vi "Stream to Image Files.vi"() -> ()   [LabVIEW 2023]
doc: "The Stream to Image Files example shows how to save images to PNG files in parallel when using a grab acquisition. Images acquired from a camera are stored in a manager and each worker loop removes an image from the manager to save to disk. When the save to disk is complete, the image is added back to the manager so it can be used to copy acquired images into again. It is recommended to use the Stream to Image Files (Optimized Performance) example if your camera settings work with a ring acquisition."
uses:
  SubVIs/Grab Manager Mode.ctl
  <vilib>/vision/driver/IMAQdx.llb/IMAQdx Buffer Number Mode.ctl
  <vilib>/Utility/High Resolution Relative Seconds.vi
  <vilib>/vision/driver/NI_Vision_Acquisition_Software.lvlib
  <resource>/objmgr/imaqdx.rc
panel:
  out "Images Acquired Per Second":dbl
  in  "Skip Count":u32
  in  "Number of Workers":u8=3 min=1 max=3
  out "Images Behind":i32
  out "Images Saved Per Second":dbl
  in  "Number of Images":u32=30
  out "Destination Folder":path
  out "Write Speed":dbl(graph) caption="Image File Write Speed"
  in  "Camera Name":refnum<k21> caption="IMAQdx Session"
  in  "Stop":bool
  # "Overview: Demonstrates how to stream images to disk in parallel when using a ring acquisition.\nRequirements: Vision Acquisition Software\nInstructions:\n1. Select the Camera Name\n2. Run the VI\n3. Reduce the Number of Workers to see if the streaming of images can keep up with fewer workers.\n4. Increase the Skip Count if Images Behind is greater than 0."
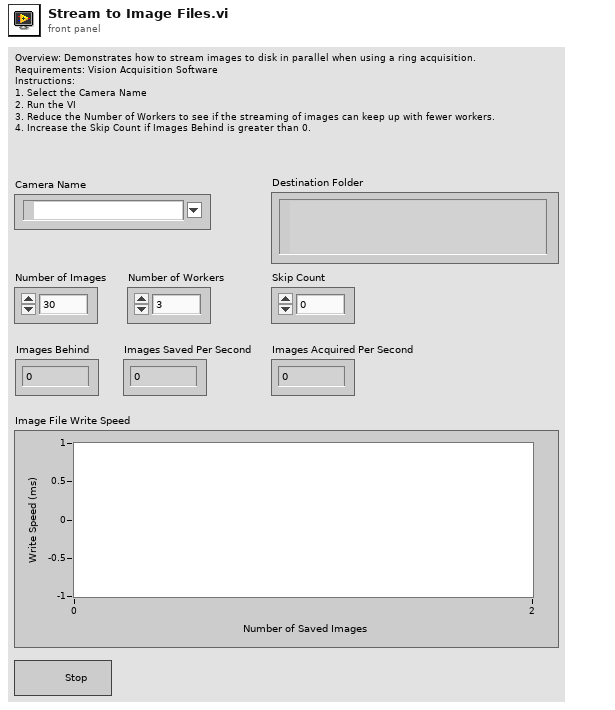
[diagram p1: front panel]
types:
  T1 = cluster{"Number of Processing Images":u32, "Image Border Size":u32}
  T2 = typedef "Grab Manager Mode.ctl" = enum16{"Create Processing Images", "Lock", "Add Acquired Image", "Get Acquired Image", "Unlock", "Dispose Processing Images"}
  T3 = typedef "IMAQdx.ctl" = refnum<k21>
  T4 = typedef "NI_Vision_Acquisition_Software.lvlib/IMAQdx Buffer Number Mode.ctl" = enum32{"Next", "Last", "Buffer Number", "Every", "Last New"}
  T5 = typedef "IMAQ Image.ctl" = refnum<image>
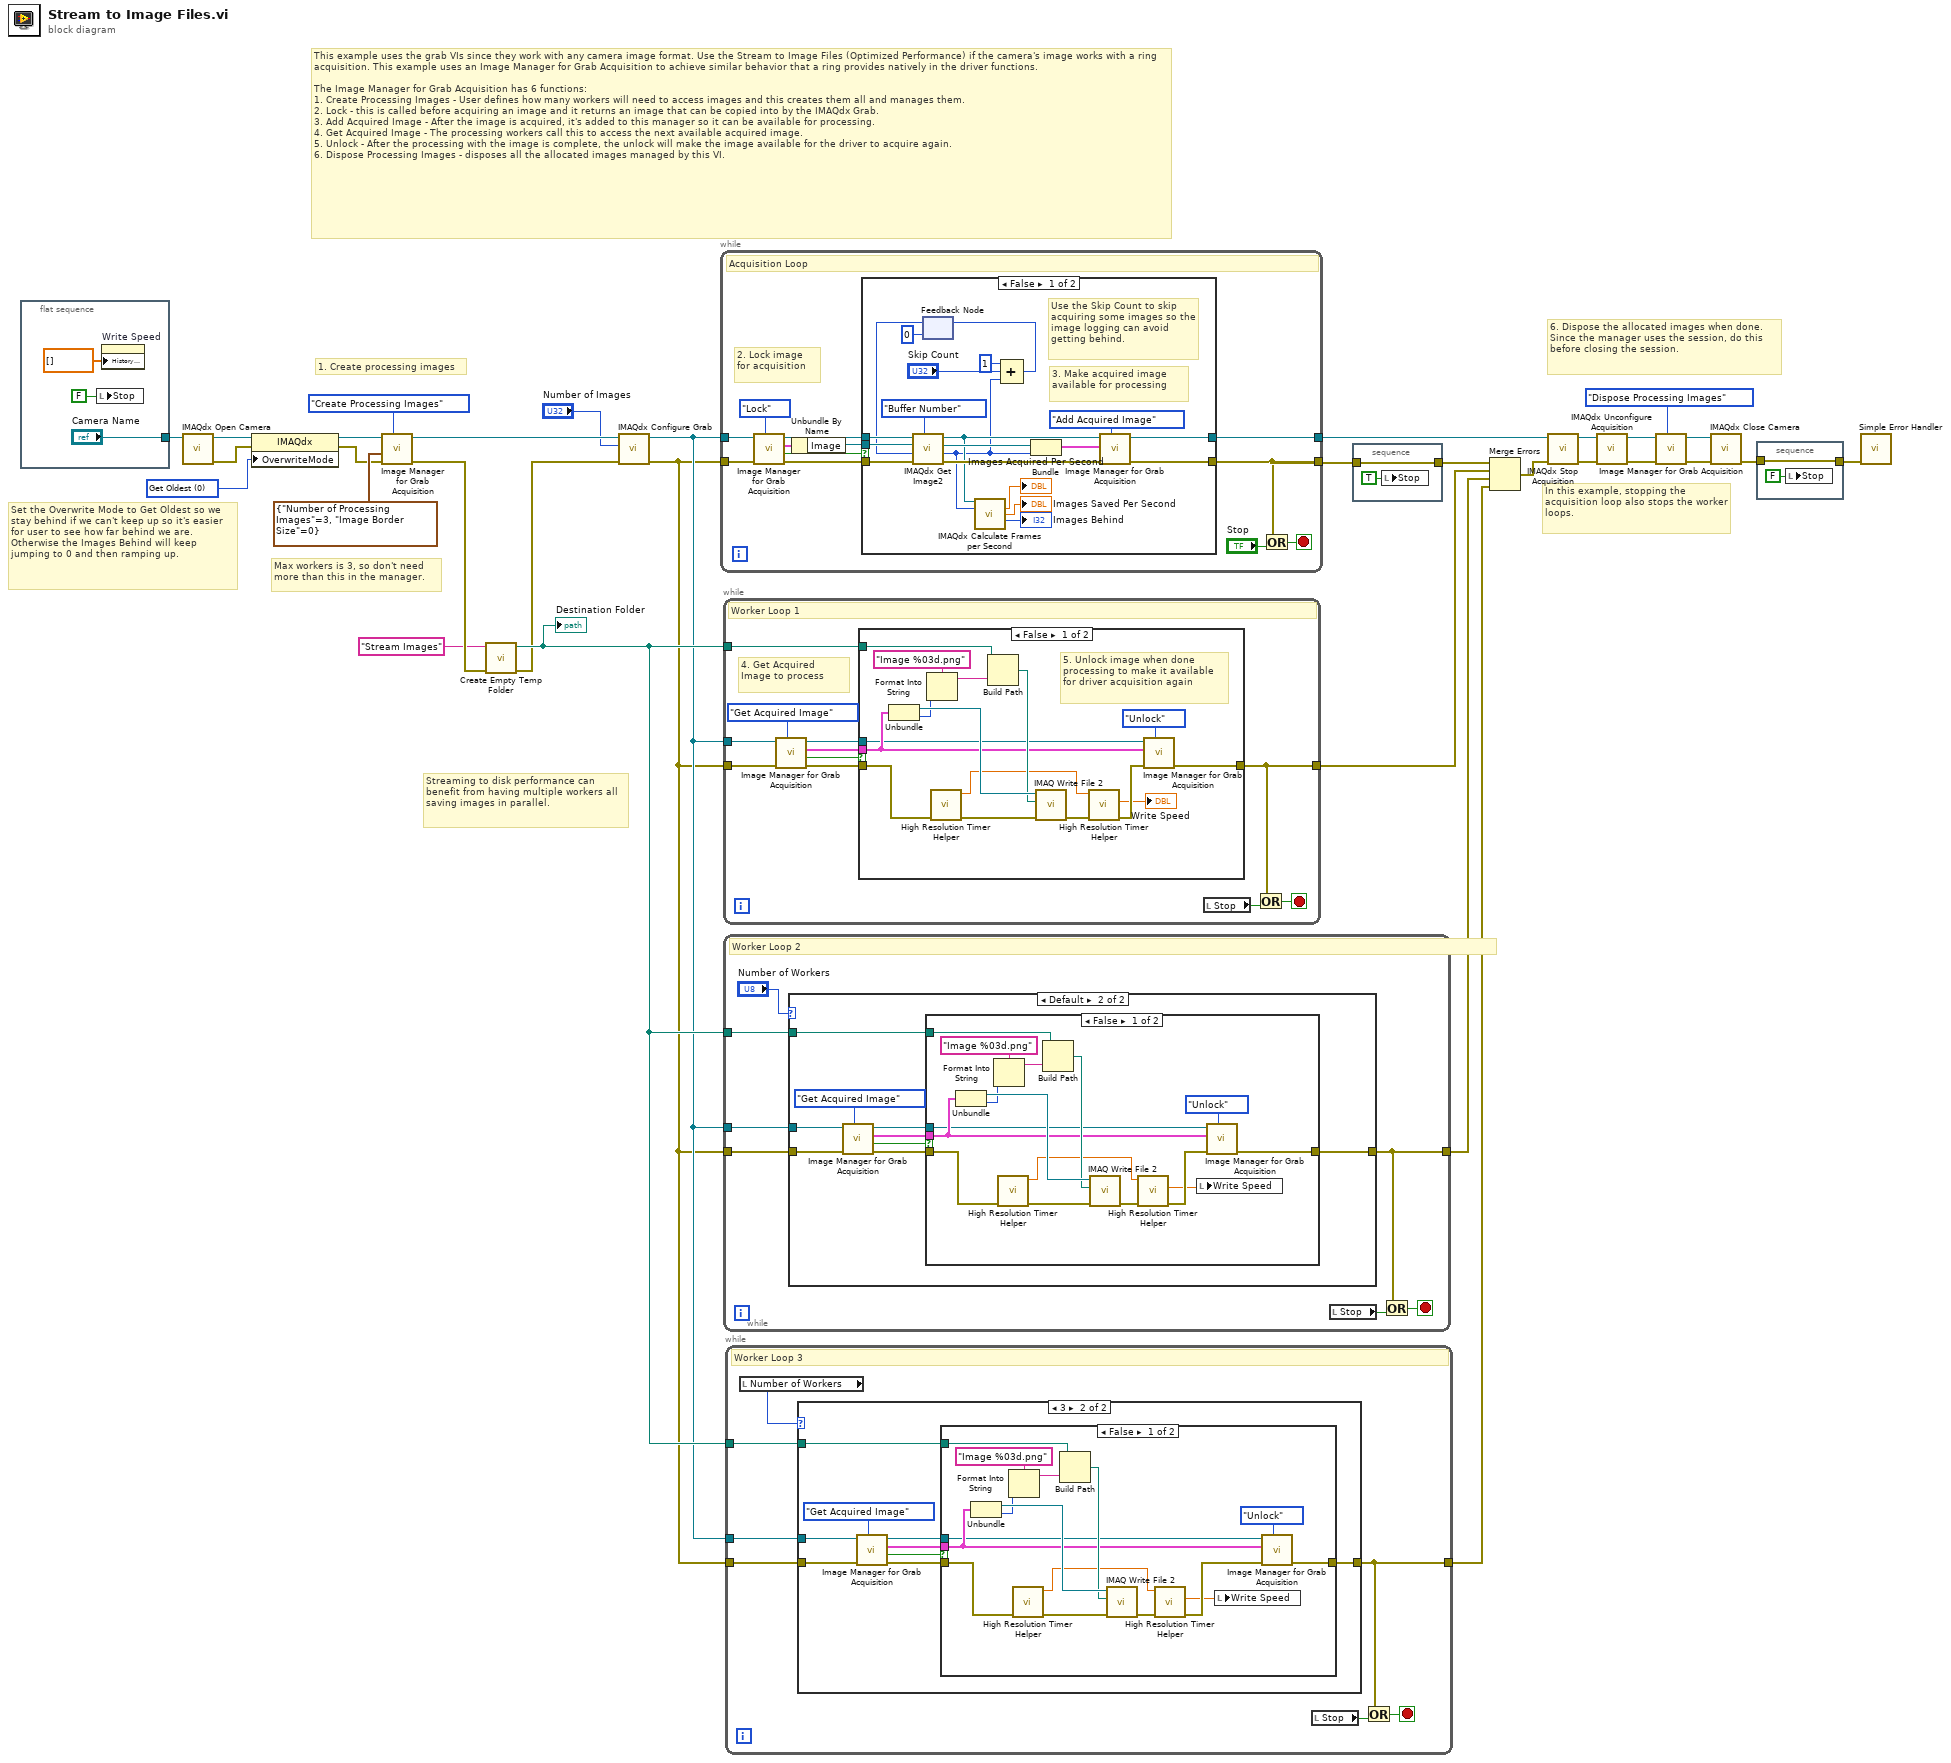
[diagram p0: block diagram]
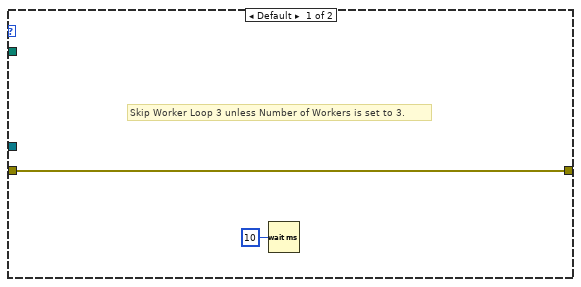
[diagram p2: hidden frame]
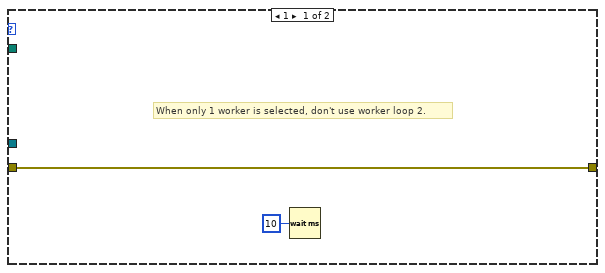
[diagram p4: hidden frame]
diagram:
  w19 = u32 0 items=["Get Oldest"=0, "Fail"=2, "Get Newest"=3] ("OverwriteMode")
  # "6. Dispose the allocated images when done. Since the manager uses the session, do this before closing the session."
  # "1. Create processing images"
  # "This example uses the grab VIs since they work with any camera image format. Use the Stream to Image Files (Optimized Performance) if the camera's image works with a ring acquisition. This example uses an Image Manager for Grab Acquisition to achieve similar behavior that a ring provides natively in the driver functions.\n\nThe Image Manager for Grab Acquisition has 6 functions:\n1. Create Processing Images - User defines how many workers will need to access images and this creates them all and manages them.\n2. Lock - this is called before acquiring an image and it returns an image that can be copied into by the IMAQdx Grab.\n3. Add Acquired Image - After the image is acquired, it's added to this manager so it can be available for processing.\n4. Get Acquired Image - The processing workers call this to access the next available acquired image.\n5. Unlock - After the processing with the image is complete, the unlock will make the image available for the driver to acquire again.\n6. Dispose Processing Images - disposes all the allocated images managed by this VI."
  # "Set the Overwrite Mode to Get Oldest so we stay behind if we can't keep up so it's easier for user to see how far behind we are. Otherwise the Images Behind will keep jumping to 0 and then ramping up."
  # "Max workers is 3, so don't need more than this in the manager."
  # "In this example, stopping the acquisition loop also stops the worker loops."
  # "Streaming to disk performance can benefit from having multiple workers all saving images in parallel."
  n1 = flat-sequence {
    tunnel: ["Camera Name"] -> w32
    frame #0 {
      n2 = local write "Stop"(FALSE ("Stop")) -> ()
      n3 = property on="Write Speed" class="WFChart (strict)"("History Data"=dbl[] []) -> ()  [unwired: 2 in, 2 out]
    }
  }
  n4 = call <vilib>:"IMAQdx Open Camera.vi"("Session In"=w32) -> ("error out"=w10:errorcluster, "Session Out"=w20:T3)  [unwired: 2 in, 7 out]
  n5 = property class="IMAQdx"(reference=w20, error in=w10, "OverwriteMode"=w19) -> (reference out=w9:T3, error out=w8:errorcluster)
  n6 = call "Image Manager for Grab Acquisition.vi"("Mode"=Grab_Manager_Mode."Create Processing Images", "error in (no error)"=w8, "Init Settings"=T1 {"Number of Processing Images"=3, "Image Border Size"=0}, "Session In"=w9) -> ("error out"=w7:errorcluster, "Session Out"=w5:T3)  [unwired: 4 in, 2 out]
  n7 = call "Create Empty Temp Folder.vi"("error in (no error)"=w7, "Folder Name"="Stream Images") -> ("error out"=w4:errorcluster, "Empty Temp Folder"=w22:path)  [unwired: 8 in]
  "Destination Folder" <- w22
  n8 = call <vilib>:"IMAQdx Configure Grab.vi"("error in"=w4, "Number of Buffers"="Number of Images", "Session In"=w5) -> ("error out"=w2:errorcluster, "Session Out"=w3:T3)  [unwired: 7 in]
  n9 = while {
    tunnel: w2 -> [w45]
    tunnel: w3 -> [w42]
    tunnel: [w43] -> w28
    tunnel: [w44] -> w27
    stop <- w46 stop-if-true
    # "2. Lock image for acquisition"
    # "Acquisition Loop"
    n10 = call "Image Manager for Grab Acquisition.vi"("Mode"=Grab_Manager_Mode."Lock", "error in (no error)"=w45, "Session In"=w42) -> ("error out"=w38:errorcluster, "No Available Image"=w39:bool, "Image Settings Out"=w37:cluster{"Image":T5, "Buffer Number":u32}, "Session Out"=w40:T3)  [unwired: 5 in]
    n11 = Unbundle By Name(w37) -> ("Image"=w36:T5)
    n12 = case shown="False" w39 {
      tunnel: [w59 w69] -> w43
      tunnel: [w58 w68] -> w44
      tunnel: w40 -> [w67 w69]
      tunnel: w38 -> [w66 w68]
      tunnel: w36 -> [w60 _]
      frame False {
        # "3. Make acquired image available for processing"
        # "Use the Skip Count to skip acquiring some images so the image logging can avoid getting behind."
        n13 = feedback #1(u32 0) -> (w49:u32)
        n14 = call <vilib>:"IMAQdx Get Image2.vi"("Buffer Number Mode (Next)"=IMAQdx_Buffer_Number_Mode."Buffer Number", "error in"=w66, "Buffer Number In"=w49, "Image In"=w60, "Session In"=w67) -> ("error out"=w62:errorcluster, "Buffer Number Out"=w53:u32, "Image Out"=w64:T5, "Session Out"=w57:T3)  [unwired: 3 in]
        n15 = call <vilib>:"IMAQdx Calculate Frames per Second.vi"("Session In"=w57, "Buffer Number"=w53) -> ("Acquired Frames per Second"=→"Images Acquired Per Second":dbl, "Processed Frames per Second"=→"Images Saved Per Second":dbl, "Images Behind"=→"Images Behind":i32)  [unwired: 7 in, 4 out]
        n16 = Compound Arithmetic op=ADD(u32 1 ("value"), "Skip Count", w53) -> (w50:u32)
        n17 = feedback-in #1(w50) -> ()
        n18 = Bundle("Image Out"=w64, "Buffer Number Out"=w53) -> (w63:cluster{"Image Out":T5, "Buffer Number Out":u32})  [unwired: 1 in]
        n19 = call "Image Manager for Grab Acquisition.vi"("Mode"=Grab_Manager_Mode."Add Acquired Image", "error in (no error)"=w62, "Image Settings In"=w63, "Session In"=w57) -> ("error out"=w58:errorcluster, "Session Out"=w59:T3)  [unwired: 4 in, 2 out]
      }
      frame True {
        # "The Lock function already has a delay inside when no images are available to prevent loop from going too fast and starving the worker threads from getting processing time."
        # "Write to disk operation is taking longer so images aren't added back to manager. Wait until there is an available image"
      }
    }
    n20 = Or(x=w44, y="Stop") -> (x .or. y?=w46:bool)
  }
  n21 = while {
    tunnel: w2 -> [w76]
    tunnel: w22 -> [w78]
    tunnel: [w77] -> w24
    tunnel: w3 -> [w71]
    stop <- w80 stop-if-true
    # "4. Get Acquired Image to process"
    # "Worker Loop 1"
    n22 = call "Image Manager for Grab Acquisition.vi"("Mode"=Grab_Manager_Mode."Get Acquired Image", "error in (no error)"=w76, "Session In"=w71) -> ("error out"=w72:errorcluster, "No Available Image"=w74:bool, "Image Settings Out"=w73:cluster{"Image":T5, "Buffer Number":u32}, "Session Out"=w70:T3)  [unwired: 5 in]
    n23 = case shown="False" w74 {
      tunnel: w72 -> [w86 w97]
      tunnel: w73 -> [w88 _]
      tunnel: [w90 w97] -> w77
      tunnel: w78 -> [w95 _]
      tunnel: w70 -> [w87 _]
      frame False {
        # "5. Unlock image when done processing to make it available for driver acquisition again"
        n24 = Unbundle(w88) -> ("Image"=w96:T5, "Buffer Number"=w92:u32)
        n25 = Format Into String(format string="Image %03d.png", w92) -> (resulting string=w94:string)  [unwired: 2 in, 1 out]
        n26 = call "High Resolution Timer Helper.vi"("error in (no error)"=w86) -> ("error out"=w85:errorcluster, "Current Time"=w82:dbl)  [unwired: 8 in, 1 out]
        n27 = Build Path(base path=w95, name or relative path=w94) -> (appended path=w91:path)
        n28 = call-poly "IMAQ Write File 2"("error in (no error)"=w85, "File Path"=w91, "Image"=w96) -> ("error out"=w84:errorcluster)  [unwired: 7 in, 1 out]
        n29 = call "High Resolution Timer Helper.vi"("error in (no error)"=w84, "Previous Time"=w82) -> ("error out"=w83:errorcluster, "Time Difference (ms)"=→"Write Speed":dbl)  [unwired: 7 in, 1 out]
        n30 = call "Image Manager for Grab Acquisition.vi"("Mode"=Grab_Manager_Mode."Unlock", "error in (no error)"=w83, "Image Settings In"=w88, "Session In"=w87) -> ("error out"=w90:errorcluster)  [unwired: 4 in, 3 out]
      }
      frame True {
        # "No acquired images to process"
      }
    }
    n31 = local read "Stop"() -> (w79:bool)
    n32 = Or(x=w77, y=w79) -> (x .or. y?=w80:bool)
  }
  n33 = while {
    tunnel: w2 -> [w100]
    tunnel: w22 -> [w101]
    tunnel: [w102] -> w23
    tunnel: w3 -> [w99]
    stop <- w104 stop-if-true
    # "Worker Loop 2"
    n34 = case shown="Default" "Number of Workers" {
      tunnel: [w106 w115] -> w102
      tunnel: w101 -> [_ w114]
      tunnel: w100 -> [w106 w110]
      tunnel: w99 -> [_ w107]
      frame 1 {
        # "When only 1 worker is selected, don't use worker loop 2."
        n35 = Wait (ms)(milliseconds to wait=u32 10) -> ()  [unwired: 1 out]
      }
      frame Default {
        n36 = call "Image Manager for Grab Acquisition.vi"("Mode"=Grab_Manager_Mode."Get Acquired Image", "error in (no error)"=w110, "Session In"=w107) -> ("error out"=w109:errorcluster, "No Available Image"=w108:bool, "Image Settings Out"=w111:cluster{"Image":T5, "Buffer Number":u32}, "Session Out"=w112:T3)  [unwired: 5 in]
        n37 = case shown="False" w108 {
          tunnel: w109 -> [w121 w132]
          tunnel: w111 -> [w123 _]
          tunnel: [w125 w132] -> w115
          tunnel: w114 -> [w130 _]
          tunnel: w112 -> [w122 _]
          frame False {
            n38 = Unbundle(w123) -> ("Image"=w131:T5, "Buffer Number"=w127:u32)
            n39 = Format Into String(format string="Image %03d.png", w127) -> (resulting string=w129:string)  [unwired: 2 in, 1 out]
            n40 = call "High Resolution Timer Helper.vi"("error in (no error)"=w121) -> ("error out"=w120:errorcluster, "Current Time"=w117:dbl)  [unwired: 8 in, 1 out]
            n41 = Build Path(base path=w130, name or relative path=w129) -> (appended path=w126:path)
            n42 = call-poly "IMAQ Write File 2"("error in (no error)"=w120, "File Path"=w126, "Image"=w131) -> ("error out"=w119:errorcluster)  [unwired: 7 in, 1 out]
            n43 = call "High Resolution Timer Helper.vi"("error in (no error)"=w119, "Previous Time"=w117) -> ("error out"=w118:errorcluster, "Time Difference (ms)"=w116:dbl)  [unwired: 7 in, 1 out]
            n44 = local write "Write Speed"(w116) -> ()
            n45 = call "Image Manager for Grab Acquisition.vi"("Mode"=Grab_Manager_Mode."Unlock", "error in (no error)"=w118, "Image Settings In"=w123, "Session In"=w122) -> ("error out"=w125:errorcluster)  [unwired: 4 in, 3 out]
          }
          frame True {
            # "No acquired images to process"
          }
        }
      }
    }
    n46 = local read "Stop"() -> (w103:bool)
    n47 = Or(x=w102, y=w103) -> (x .or. y?=w104:bool)
  }
  n48 = while {
    tunnel: w2 -> [w136]
    tunnel: w22 -> [w137]
    tunnel: [w134] -> w21
    tunnel: w3 -> [w135]
    stop <- w139 stop-if-true
    # "Worker Loop 3"
    n49 = local read "Number of Workers"() -> (w133:u8)
    n50 = case shown="3" w133 {
      tunnel: w137 -> [_ w150]
      tunnel: w136 -> [w141 w149]
      tunnel: w135 -> [_ w148]
      tunnel: [w141 w142] -> w134
      frame Default {
        # "Skip Worker Loop 3 unless Number of Workers is set to 3."
        n51 = Wait (ms)(milliseconds to wait=u32 10) -> ()  [unwired: 1 out]
      }
      frame 3 {
        n52 = call "Image Manager for Grab Acquisition.vi"("Mode"=Grab_Manager_Mode."Get Acquired Image", "error in (no error)"=w149, "Session In"=w148) -> ("error out"=w144:errorcluster, "No Available Image"=w145:bool, "Image Settings Out"=w146:cluster{"Image":T5, "Buffer Number":u32}, "Session Out"=w147:T3)  [unwired: 5 in]
        n53 = case shown="False" w145 {
          tunnel: w144 -> [w156 w167]
          tunnel: w146 -> [w158 _]
          tunnel: [w160 w167] -> w142
          tunnel: w150 -> [w165 _]
          tunnel: w147 -> [w157 _]
          frame False {
            n54 = Unbundle(w158) -> ("Image"=w166:T5, "Buffer Number"=w162:u32)
            n55 = Format Into String(format string="Image %03d.png", w162) -> (resulting string=w164:string)  [unwired: 2 in, 1 out]
            n56 = call "High Resolution Timer Helper.vi"("error in (no error)"=w156) -> ("error out"=w155:errorcluster, "Current Time"=w152:dbl)  [unwired: 8 in, 1 out]
            n57 = Build Path(base path=w165, name or relative path=w164) -> (appended path=w161:path)
            n58 = call-poly "IMAQ Write File 2"("error in (no error)"=w155, "File Path"=w161, "Image"=w166) -> ("error out"=w154:errorcluster)  [unwired: 7 in, 1 out]
            n59 = call "High Resolution Timer Helper.vi"("error in (no error)"=w154, "Previous Time"=w152) -> ("error out"=w153:errorcluster, "Time Difference (ms)"=w151:dbl)  [unwired: 7 in, 1 out]
            n60 = local write "Write Speed"(w151) -> ()
            n61 = call "Image Manager for Grab Acquisition.vi"("Mode"=Grab_Manager_Mode."Unlock", "error in (no error)"=w153, "Image Settings In"=w158, "Session In"=w157) -> ("error out"=w160:errorcluster)  [unwired: 4 in, 3 out]
          }
          frame True {
            # "No acquired images to process"
          }
        }
      }
    }
    n62 = local read "Stop"() -> (w138:bool)
    n63 = Or(x=w134, y=w138) -> (x .or. y?=w139:bool)
  }
  n64 = stacked-sequence {
    tunnel: [w168] -> w26
    tunnel: w27 -> [w168]
    frame #0 {
      n65 = local write "Stop"(TRUE ("Stop")) -> ()
    }
  }
  n66 = Merge Errors(w26, w24, w23, w21) -> (w29:errorcluster)
  n67 = call <vilib>:"IMAQdx Stop Acquisition.vi"("error in"=w29, "Session In"=w28) -> ("error out"=w30:errorcluster, "Session Out"=w31:T3)  [unwired: 8 out]
  n68 = call <vilib>:"IMAQdx Unconfigure Acquisition.vi"("error in"=w30, "Session In"=w31) -> ("error out"=w17:errorcluster, "Session Out"=w18:T3)  [unwired: 8 out]
  n69 = call "Image Manager for Grab Acquisition.vi"("Mode"=Grab_Manager_Mode."Dispose Processing Images", "error in (no error)"=w17, "Session In"=w18) -> ("error out"=w14:errorcluster, "Session Out"=w15:T3)  [unwired: 5 in, 2 out]
  n70 = call <vilib>:"IMAQdx Close Camera.vi"("error in"=w14, "Session In"=w15) -> ("error out"=w13:errorcluster)  [unwired: 9 out]
  n71 = stacked-sequence {
    tunnel: [w170] -> w25
    tunnel: w13 -> [w170]
    frame #0 {
      n72 = local write "Stop"(FALSE ("Stop")) -> ()
    }
  }
  n73 = call <vilib>:"Simple Error Handler.vi"("error in (no error)"=w25) -> ()  [unwired: 4 in, 5 out]
